vi "Get TXP Measurement Parameters.vi"(8 "error in (no error)":errorcluster, 11 "niDTS BT INSTR TX in":refnum<class "niDTS BT INSTR TX.lvclass">) -> (0 "error out":errorcluster, 2 "TXP Measurement Parameters":T1={"TXP Power Enable"=FALSE, "TXP Averages"=1, "Averaging Type"=enum."RMS"}, 3 "niDTS BT INSTR TX out":refnum<class "niDTS BT INSTR TX.lvclass">)   [LabVIEW 2015, in "niDTS BT.lvlib" / "niDTS BT INSTR TX.lvclass"]
uses:
  niDTS BT INSTR TX.lvclass
  Includes/niDTS BT INC TXP Measurement Parameters.ctl
  niDTS BT INSTR TX.lvclass/niDTS BT INSTR TX.ctl
  niDTS BT.lvlib
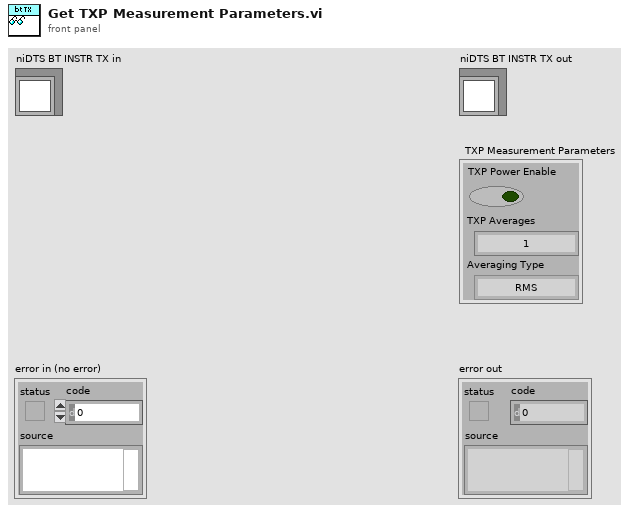
[diagram p1: front panel]
types:
  T1 = typedef "niDTS BT.lvlib/niDTS BT INC TXP Measurement Parameters.ctl" = cluster{"TXP Power Enable":bool, "TXP Averages":i32, "Averaging Type":enum16{"RMS", "LOG", "SCALAR", "MAX", "MIN"}}
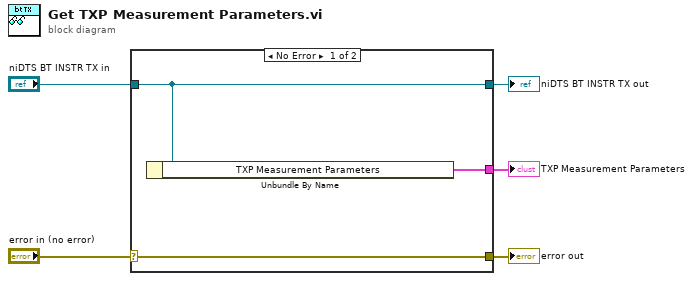
[diagram p0: block diagram]
diagram:
  n1 = case shown="No Error" "error in (no error)" {
    selector: "error in (no error)" -> [w8 w9]
    tunnel: [w8 w9] -> w4
    tunnel: [w7 w10] -> w2
    tunnel: "niDTS BT INSTR TX in" -> [w7 w10]
    tunnel: [w6 _] -> w1
    frame No Error {
      n2 = Unbundle By Name(w7) -> ("TXP Measurement Parameters"=w6:T1)
    }
    frame Error {
    }
  }
  "error out" <- w4
  "niDTS BT INSTR TX out" <- w2
  "TXP Measurement Parameters" <- w1
